vi "CSM - Global Log Queue.vi"(8 "Error In":errorcluster caption="error in (no error)") -> (0 "error out":errorcluster, 3 "Global Log Queue":refnum<queue>)   [LabVIEW 2017, in "Communicable State Machine.lvlib"]
doc: "Obtains the global log queue refnum. Global log events can be retrieved from this queue.\n\n\n> [!NOTE] <b>CSM Global Log Functionality</b>\n>\n> The CSM Global Log functionality is used to view global log change events, serving scenarios such as debugging and monitoring.\n> The following is the information that can be logged:\n> - Module state modifications\n> - Inter-module message communication, including data returns\n> - Message completion records of asynchronous and synchronous messages, `AsyncMsg Complete` and `SyncMsg Complete`, which carry the response\n> - Module status publishing\n> - Module creation and destruction\n> - Module state registration and unregistration\n> - Error information handled by modules\n> - User-defined events\n>\n> Debugging tools are primarily developed based on the Global Log API. You can develop debugging tools according to your own needs.\n\n\n> [!NOTE] <b>CSM Global Log Acquisition Methods</b>\n>\n> CSM provides two methods for acquiring global logs: Queue and Event. The Queue processing method is recommended because the queue interface is more efficient and offers greater flexibility in selecting log processing schemes based on the number of accumulated logs in the queue.\n\n\n<b>Reference Examples</b>:\n- `4. Advance Examples\\Filter From Source(Queue).vi`\n- `4. Advance Examples\\Filter From Subscriber(Queue).vi`\n\n-- <b>Indicators</b> --\n- <b>Global Log Queue</b>: Global log queue refnum."
uses:
  Communicable State Machine.lvlib
  _Support/Typedef/_CSM_GlobalLog_MSG.ctl
  _Support/Typedef/_CSM_Response Source Message.ctl
  _Support/Typedef/_CSM_GlobalLog_MSG_TYPE.ctl
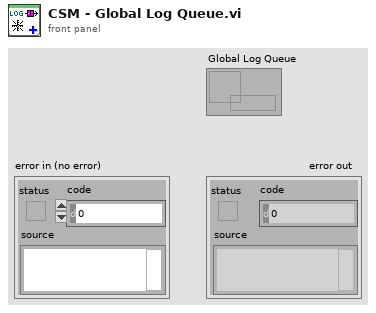
[diagram p1: front panel]
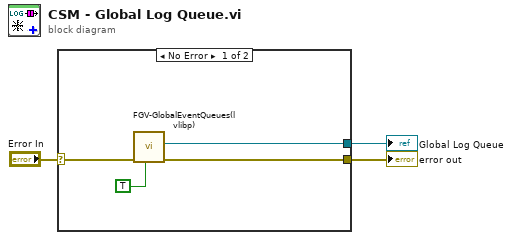
[diagram p0: block diagram]
diagram:
  n1 = case shown="No Error" "Error In" {
    selector: "Error In" -> [w7 w8]
    tunnel: [w6 w8] -> w3
    tunnel: [w5 _] -> w1
    frame No Error {
      n2 = call "FGV-GlobalEventQueues(lvlibp).vi"("Create? (F)"=TRUE ("Create(F)"), "error in (no error)"=w7) -> ("error out"=w6:errorcluster, "CreatedQueue"=w5:refnum<queue>)  [unwired: 7 in, 1 out]
    }
    frame Error {
    }
  }
  "error out" <- w3
  "Global Log Queue" <- w1
